vi "StringifiedData.vi"(8 "error in (no error)":errorcluster, 11 "Message in":refnum<class "Message.lvclass">) -> (0 "error out":errorcluster, 2 "Stringified Data":string, 3 "Message out":refnum<class "Message.lvclass">)   [LabVIEW 2013, in "LapDog.Messaging.v3.lvlib" / "Message.lvclass"]
doc: "This VI is used for the message probe. Child classes may override it and provide the message data in string format or a short string describing the data the message contains. This string will be displayed in the probe window."
uses:
  Message.lvclass
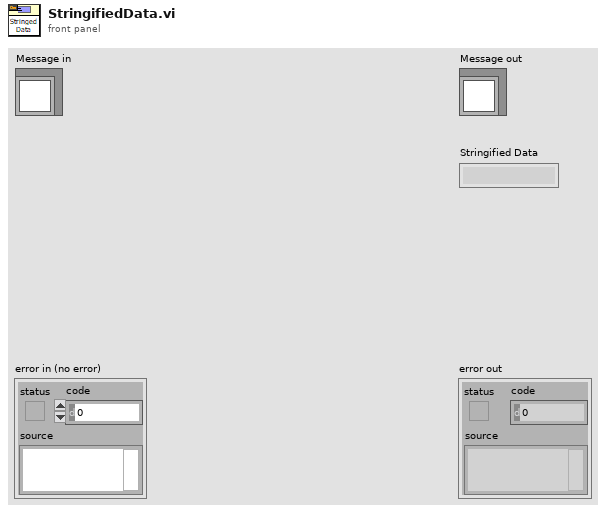
[diagram p1: front panel]
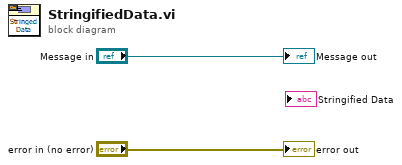
[diagram p0: block diagram]
diagram:
  "error out" <- "error in (no error)"
  "Message out" <- "Message in"
